vi "VNA - Minor Cal Dual Port.vi"(8 "error in":errorcluster {"code" format="%.0x"}, 9 "file path":path=path "C:/Calibration Files/CK Calibration - MEMS_SWITCH_50MHz.chx", 10 "port":string="port1", 11 "resource name":refnum<k15>="5632_0") -> (0 "error out":errorcluster {"code" format="%.0x"}, 1 "init cal state":i32(ring) items=["Uncalibrated", "Calibrating", "Calibrated"], 5 "P1 Time":dbl, 7 "P1 Distance":dbl)   [LabVIEW 2013]
uses:
  <instrlib>/niVNA/niVNA.llb/niVNA Load Calibration And Configuration Data From File.vi
  <instrlib>/niVNA/niVNA.llb/niVNA Save Calibration And Configuration Data To File.vi
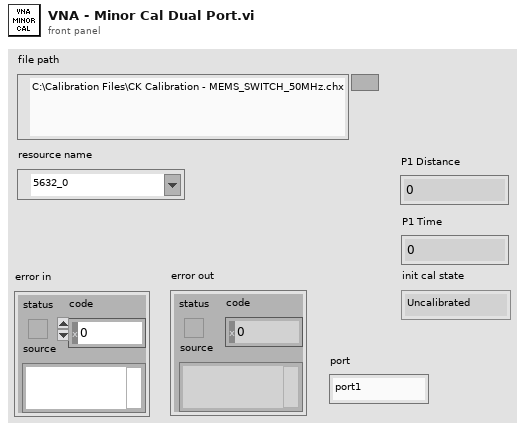
[diagram p1: front panel]
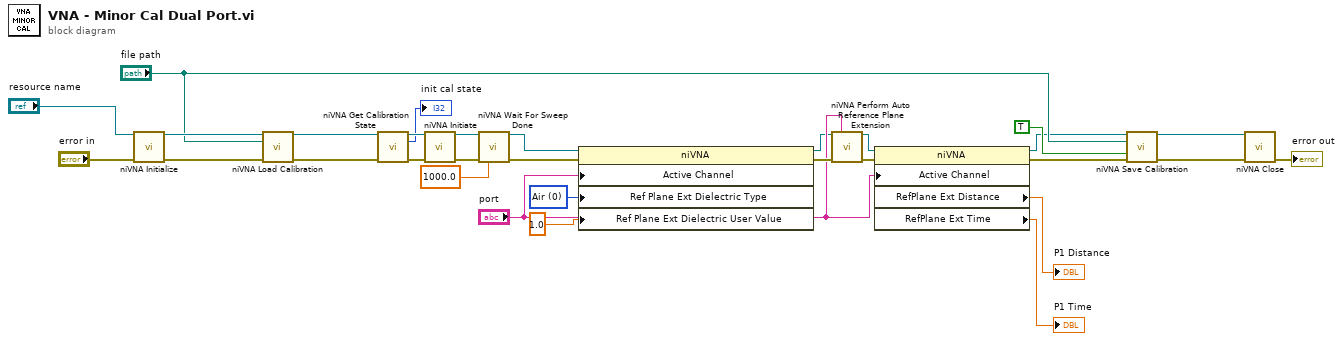
[diagram p0: block diagram]
diagram:
  w12 = 0 items=["Air", "Polyethylene", "Teflon", "Micro Teflon", "User Value"] ("Test Signal:Ref Plane Extension:Dielectric Type")
  n1 = call <instrlib>:"niVNA Initialize.vi"("resource name"="resource name", "error in"="error in") -> ("instrument handle"=w22:refnum<k15>, "error out"=w28:errorcluster)  [unwired: 12 in]
  n2 = call-poly <instrlib>:"niVNA Load Calibration.vi"("instrument handle"=w22, "file path"="file path", "error in"=w28) -> ("instrument handle out"=w21:refnum<k15>, "error out"=w27:errorcluster)  [unwired: 11 in]
  n3 = call <instrlib>:"niVNA Get Calibration State.vi"("instrument handle"=w21, "error in"=w27) -> ("instrument handle out"=w20:refnum<k15>, "state"=→"init cal state":i32, "error out"=w26:errorcluster)  [unwired: 11 in]
  n4 = call <instrlib>:"niVNA Initiate.vi"("instrument handle"=w20, "error in"=w26) -> ("instrument handle out"=w19:refnum<k15>, "error out"=w25:errorcluster)  [unwired: 12 in]
  n5 = call <instrlib>:"niVNA Wait For Sweep Done.vi"("instrument handle"=w19, "error in"=w25, "timeout"=1000.0) -> ("instrument handle out"=w2:refnum<k15>, "error out"=w5:errorcluster)  [unwired: 11 in]
  n6 = property class="niVNA"(reference=w2, error in=w5, "Active Channel"="port", "Ref Plane Ext Dielectric Type"=w12, "Ref Plane Ext Dielectric User Value"=1.0 ("Test Signal:Ref Plane Extension:Time")) -> (reference out=w4:refnum<k15>, error out=w15:errorcluster)
  n7 = call <instrlib>:"niVNA Perform Auto Reference Plane Extension.vi"("instrument handle"=w4, "port"="port", "error in"=w15) -> ("instrument handle out"=w1:refnum<k15>, "error out"=w6:errorcluster)  [unwired: 11 in]
  n8 = property class="niVNA"(reference=w1, error in=w6, "Active Channel"="port") -> (reference out=w7:refnum<k15>, error out=w3:errorcluster, "RefPlane Ext Distance"=→"P1 Distance":dbl, "RefPlane Ext Time"=→"P1 Time":dbl)
  n9 = call-poly <instrlib>:"niVNA Save Calibration.vi"("instrument handle"=w7, "file path"="file path", "overwrite"=TRUE, "error in"=w3) -> ("instrument handle out"=w18:refnum<k15>, "error out"=w24:errorcluster)  [unwired: 10 in]
  n10 = call <instrlib>:"niVNA Close.vi"("instrument handle"=w18, "error in"=w24) -> ("error out"=→"error out":errorcluster)  [unwired: 13 in]
